vi "Temp konwersja.vi"(7 "Konwersja (stC ->K)":enum16{"Brak", "stC -> K", "K -> stC"}(ring)=enum."stC -> K", 8 "error in (no error)":errorcluster, 10 "Temp in (0)":dbl) -> (0 "error out":errorcluster, 2 "Temp out":dbl)   [LabVIEW 2014]
doc: "Konwertuje wartoœci temperatury miêdzy ró¿nymi skalami"
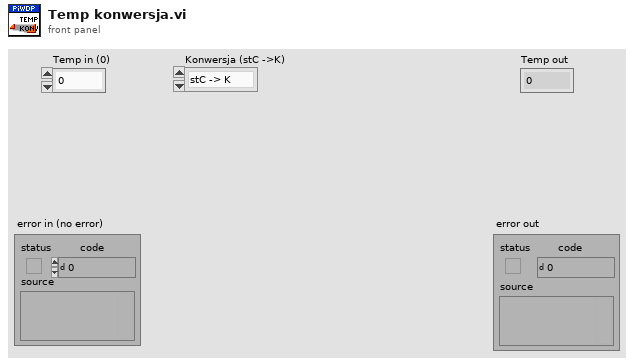
[diagram p1: front panel]
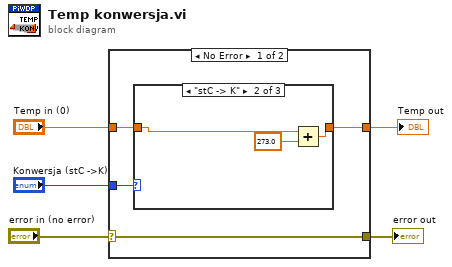
[diagram p0: block diagram]
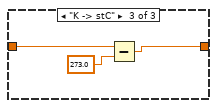
[diagram p3: hidden frame]
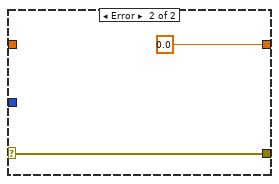
[diagram p4: hidden frame]
diagram:
  n1 = case shown="No Error" "error in (no error)" {
    selector: "error in (no error)" -> [w8 w18]
    tunnel: [w8 w18] -> w4
    tunnel: "Konwersja (stC ->K)" -> [w9 _]
    tunnel: "Temp in (0)" -> [w7 _]
    tunnel: [w6 0.0 ("Temp in")] -> w1
    frame No Error {
      n2 = case shown="\"stC -> K\"" w9 {
        tunnel: w7 -> [w10 w13 w16]
        tunnel: [w10 w12 w14] -> w6
        frame "Brak", Default {
        }
        frame "stC -> K" {
          n3 = Add(x=w13, y=273.0) -> (x+y=w12:dbl)
        }
        frame "K -> stC" {
          n4 = Subtract(x=w16, y=273.0) -> (x-y=w14:dbl)
        }
      }
    }
    frame Error {
    }
  }
  "error out" <- w4
  "Temp out" <- w1
